vi "Check Loop Error.vi"(7 "Error MHL Name (\"Error\")":string="Error", 10 "ErrorIn":errorcluster, 11 "Ignore Errors":i32[](array[numeric])) -> (2 "Queued?":bool)   [LabVIEW 2020, in "main.lvlib"]
doc: "Check Loop Error and enqueue to MHL Loop"
uses:
  main.lvlib
panel:
  # "Description\n\nCheck Loop Error and enqueue to MHL Loop"
  # "INPUTS"
  # "OUTPUTS"
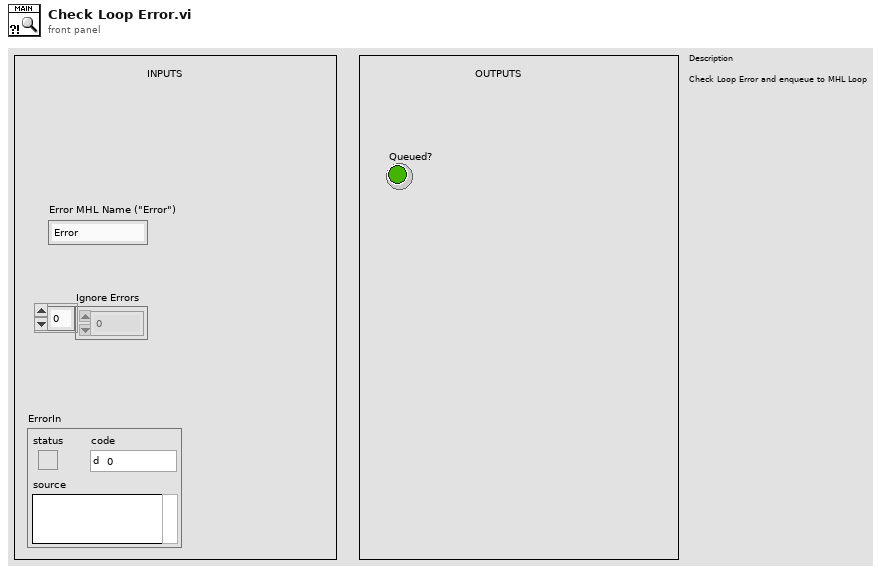
[diagram p1: front panel]
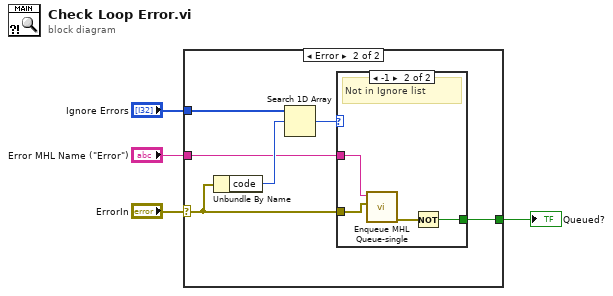
[diagram p0: block diagram]
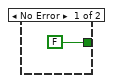
[diagram p2: hidden frame]
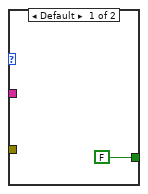
[diagram p3: hidden frame]
diagram:
  n1 = case shown="Error" "ErrorIn" {
    selector: "ErrorIn" -> [_ w6]
    tunnel: "Ignore Errors" -> [_ w10]
    tunnel: [FALSE w8] -> w2
    tunnel: "Error MHL Name (\"Error\")" -> [_ w7]
    frame No Error {
    }
    frame Error {
      n2 = Unbundle By Name(w6) -> ("code"=w11:i32)
      n3 = Search 1D Array(1D array=w10, element=w11) -> (index of element=w9:i32)  [unwired: 1 in]
      n4 = case shown="-1" w9 {
        tunnel: [FALSE w15] -> w8
        tunnel: w7 -> [_ w14]
        tunnel: w6 -> [_ w13]
        frame Default {
        }
        frame -1 {
          # "Not in Ignore list"
          n5 = call "Enqueue MHL Queue-single.vi"("Data"=w13, "Command"=w14) -> ("ErrorOut"=w16:errorcluster)  [unwired: 9 in]
          n6 = Not(x=w16) -> (.not. x?=w15:bool)
        }
      }
    }
  }
  "Queued?" <- w2
